vi "GetControlRefByPath.vi"(0 "VI Reference In":refnum<vi>, 1 "delimiter (>>)":string, 7 "Control Path":string, 11 "error In":errorcluster) -> (4 "VI Reference Out":refnum<vi>, 8 "Ctl Refnum":refnum<vi>, 15 "error out":errorcluster)   [LabVIEW 2016]
doc: "<b>Gives the reference of controls in other VI.</b>\n\nThe path of the control should be given in the successive index of the array"
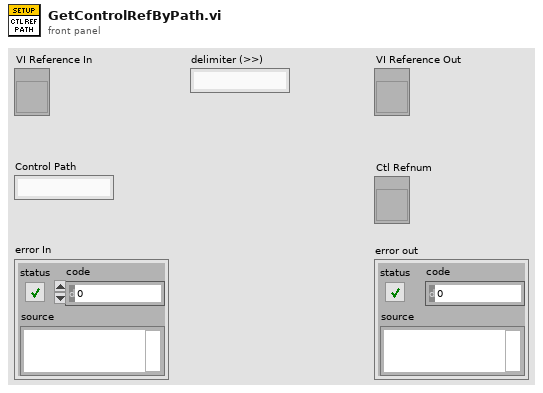
[diagram p1: front panel]
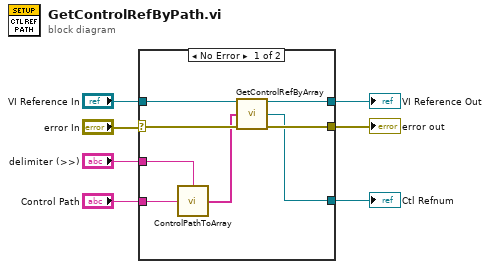
[diagram p0: block diagram]
diagram:
  n1 = case shown="No Error" "error In" {
    selector: "error In" -> [w15 w17]
    tunnel: "Control Path" -> [w10 _]
    tunnel: [w14 w17] -> w6
    tunnel: [w11 _] -> w5
    tunnel: "VI Reference In" -> [w13 w16]
    tunnel: [w12 w16] -> w2
    tunnel: "delimiter (>>)" -> [w8 _]
    frame No Error {
      n2 = call "ControlPathToArray.vi"("Control Name"=w10, "delimiter (>>)"=w8) -> ("Array"=w9:string[])
      n3 = call "GetControlRefByArray.vi"("VI Reference In"=w13, "Control Path"=w9, "error In"=w15) -> ("VI Reference Out"=w12:refnum<vi>, "Ctl Refnum"=w11:refnum<vi>, "error out"=w14:errorcluster)  [unwired: 10 in]
    }
    frame Error {
    }
  }
  "Ctl Refnum" <- w5
  "error out" <- w6
  "VI Reference Out" <- w2
